vi "Write State.vi"(8 "error in (no error)":errorcluster, 10 "new state":string, 11 "Communication Channel in":refnum<class "Communication Channel.lvclass">) -> (0 "error out":errorcluster, 3 "Communication Channel out":refnum<class "Communication Channel.lvclass">)   [LabVIEW 2018, in "Communication Channel.lvclass"]
uses:
  Communication Channel.lvclass
  Communication Channel.lvclass/Communication Channel.ctl
  State Machine/State Machine.lvclass
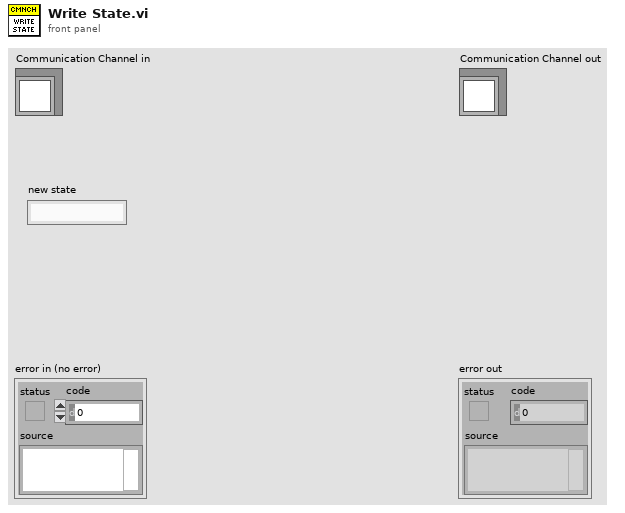
[diagram p1: front panel]
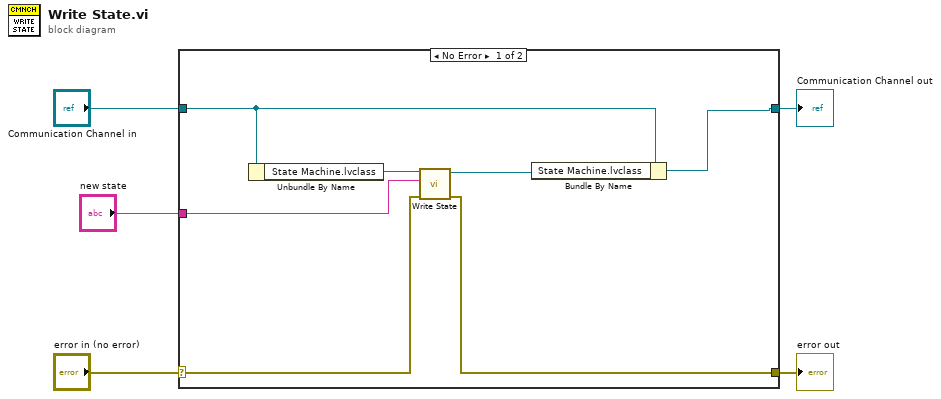
[diagram p0: block diagram]
diagram:
  n1 = case shown="No Error" "error in (no error)" {
    selector: "error in (no error)" -> [w7 w14]
    tunnel: [w6 w14] -> w4
    tunnel: [w10 w13] -> w2
    tunnel: "Communication Channel in" -> [w11 w13]
    tunnel: "new state" -> [w8 _]
    frame No Error {
      n2 = Unbundle By Name(w11) -> ("State Machine.lvclass"=w12:refnum<class "State Machine.lvclass">)
      n3 = call-dynamic "Write State.vi"("error in (no error)"=w7, "State"=w8, "State Machine in"=w12) -> ("error out"=w6:errorcluster, "State Machine out"=w9:refnum<class "State Machine.lvclass">)  [unwired: 7 in]
      n4 = Bundle By Name(cluster=w11, "State Machine.lvclass"=w9) -> (w10:refnum<class "Communication Channel.lvclass">)
    }
    frame Error {
    }
  }
  "error out" <- w4
  "Communication Channel out" <- w2
